vi "LEP_RV_GenerateBoardHeader.vi"(6 "Config":T1={"Enable debugging"=FALSE, "Debug Options"=0, "Use stack variables"=FALSE, "Generate serial only"=FALSE, "Generate guard code"=FALSE, "Generate Integer Only"=FALSE, "Generate C Function Calls"=TRUE, "ExpressionFolding"=TRUE, "Constant Allocation"=0, "Constant Deallocation"=0, "Build Specification ID"="", "Preprocessor symbols (define)"="", "Compiler Flags"="", "Linker Flags"="", "Mode"=1, "Optimization"=1, "Optimize for time"=FALSE, "Enable cross-module optimization"=FALSE, "Include paths"=[], "Optimize heap size"=TRUE, "Use MicroLib"=FALSE, "Debug Mode"=2, "Enable profile information"=FALSE, "Host name"="board", "Use DHCP"=TRUE, "IP address"="0.0.0.0", "Subnet mask"="", "Gateway"="0.0.0.0", "Primary DNS"="0.0.0.0", "Secondary DNS"="0.0.0.0", "MAC in target memory"=TRUE, "MAC address"="", "Console output"=1, "Target serial port"=1} {"Constant Deallocation" items=["Out of Scope", "VI End", "Application End"]; "Constant Allocation" items=["First Use", "Containing Loop", "VI Initialization", "Application Initialization"]; "Target serial port" items=["0", "1", "2", "3"]; "Console output" items=["Processor status window", "Serial port"]; "Optimization" items=["Level 0 (-O0)", "Level 1 (-O1)", "Level 2 (-O2)", "Level 3 (-O3)"]; "Mode" items=["ARM-Mode", "Thumb-Mode"]; "Debug Options" items=["Use ULINK Debugger", "Use Simulator"]; "Debug Mode" items=["Instrumented (serial port)", "Instrumented (TCP/IP)", "Non-instrumented (JTAG/USB)"]}, 8 "error in (no error)":errorcluster, 9 "Build Path":path=path "C:/ni/RealView Hello World/RealView", 11 "Rebuild":bool) -> (0 "error out":errorcluster)   [LabVIEW 2011]
doc: "Runs the embedded application on a console located in the <B>Build Path</B> directory ."
uses:
  LEP_RV_Config.ctl
  <vilib>/Platform/EmbProject/Plugins/utilities/LEP_Utilities_GetSetProjectData_U32.vi
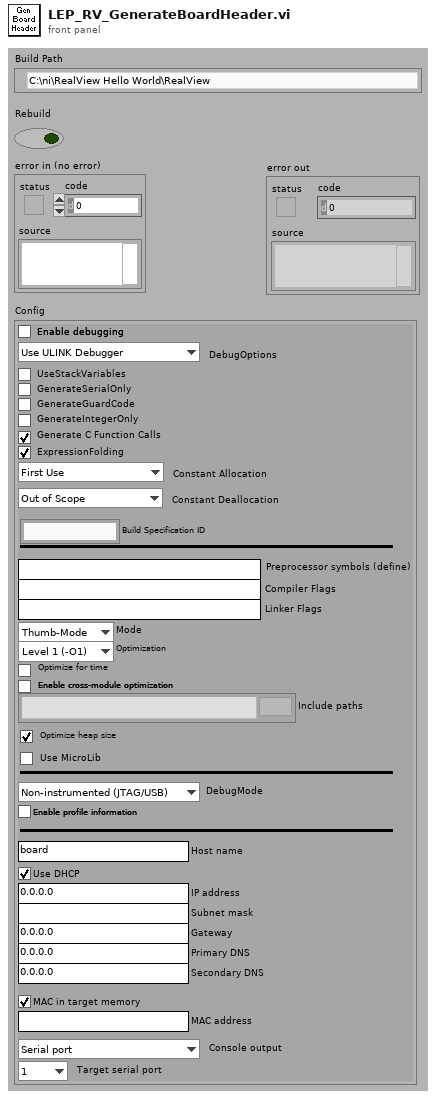
[diagram p1: front panel]
types:
  T1 = typedef "LEP_RV_Config.ctl" = cluster{"Enable debugging":bool, "Debug Options":u16, "Use stack variables":bool, "Generate serial only":bool, "Generate guard code":bool, "Generate Integer Only":bool, "Generate C Function Calls":bool, "ExpressionFolding":bool, "Constant Allocation":u16, "Constant Deallocation":u16, "Build Specification ID":string, "Preprocessor symbols (define)":string, "Compiler Flags":string, "Linker Flags":string, "Mode":u16, "Optimization":u16, "Optimize for time":bool, "Enable cross-module optimization":bool, "Include paths":path[], "Optimize heap size":bool, "Use MicroLib":bool, "Debug Mode":u16, "Enable profile information":bool, "Host name":string, "Use DHCP":bool, "IP address":string, "Subnet mask":string, "Gateway":string, "Primary DNS":string, "Secondary DNS":string, "MAC in target memory":bool, "MAC address":string, "Console output":u16, "Target serial port":u16}
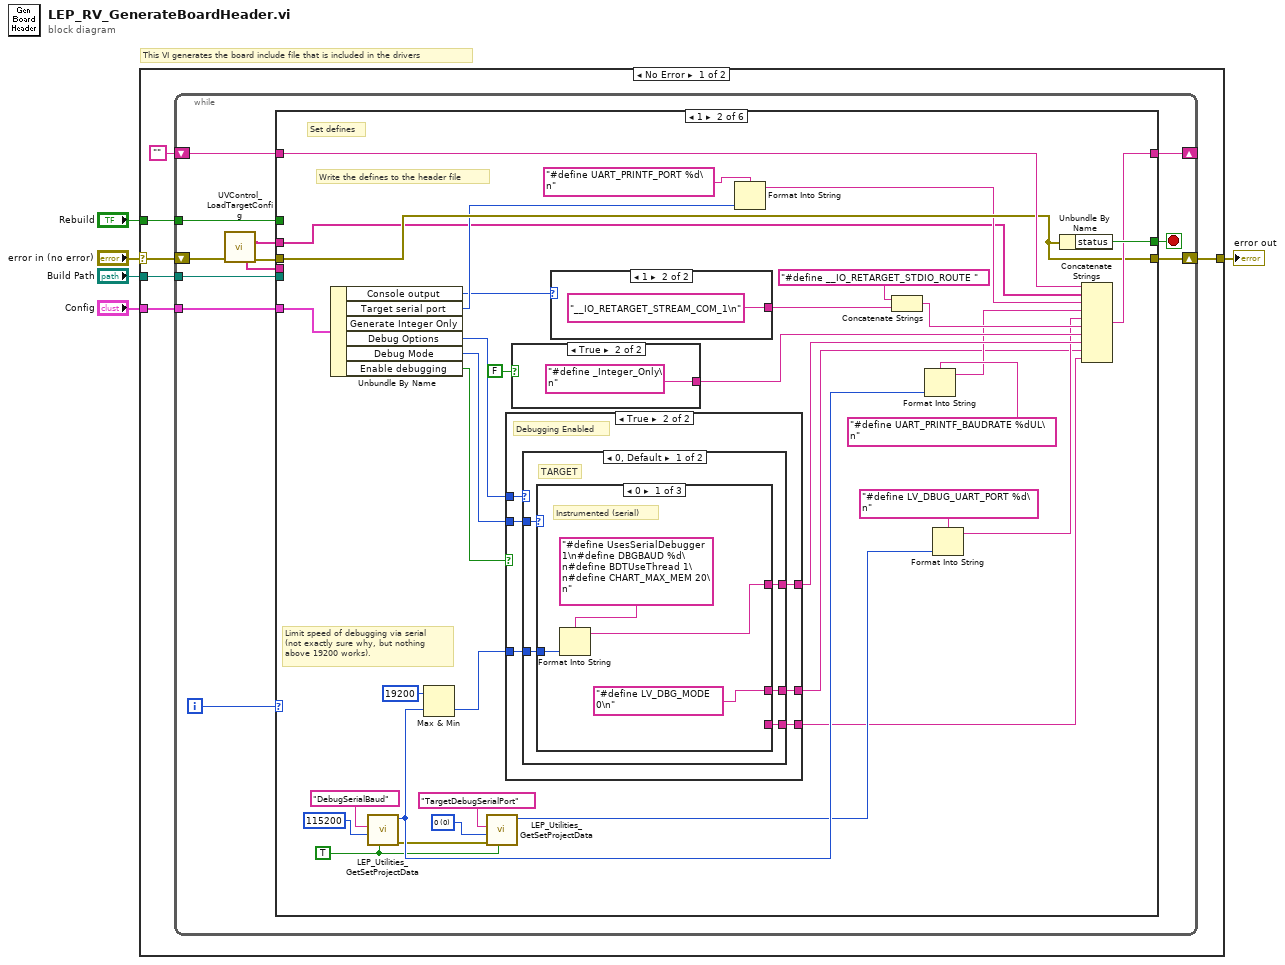
[diagram p0: block diagram]
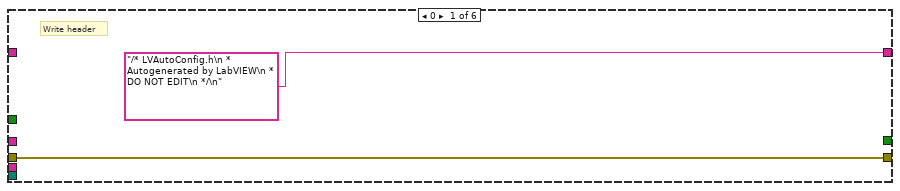
[diagram p2: hidden frame]
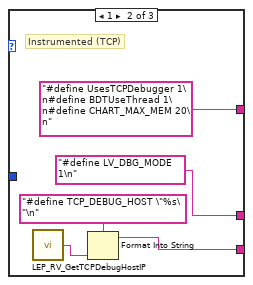
[diagram p4: hidden frame]
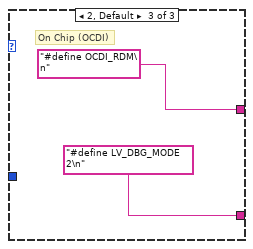
[diagram p5: hidden frame]
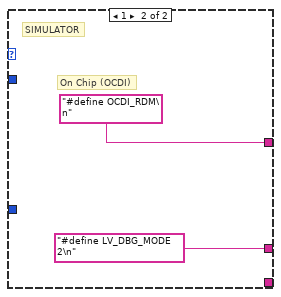
[diagram p6: hidden frame]
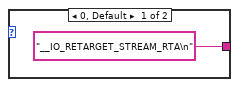
[diagram p7: hidden frame]
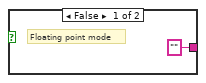
[diagram p8: hidden frame]
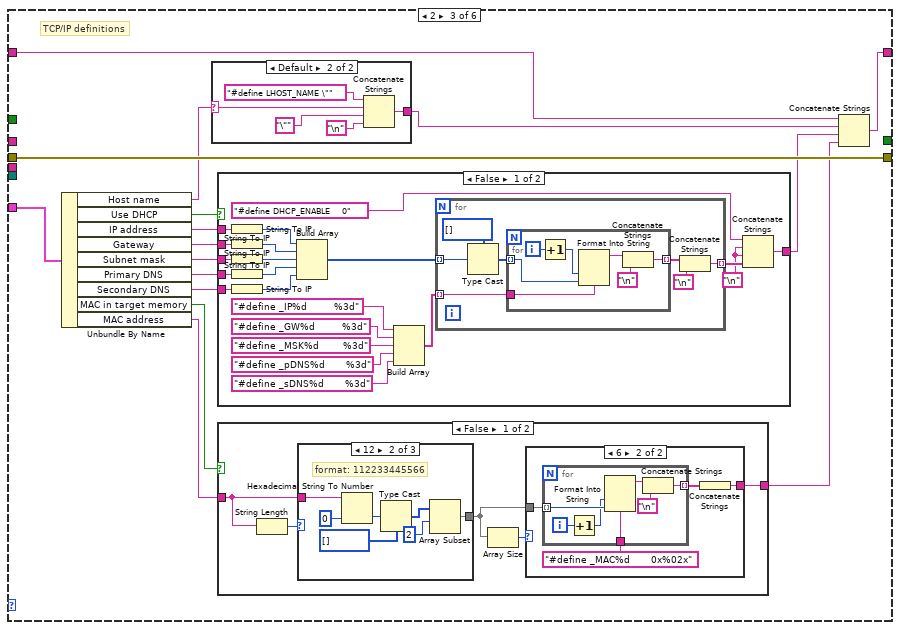
[diagram p9: hidden frame]
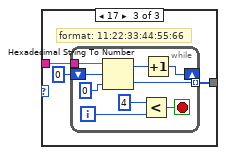
[diagram p11: hidden frame]
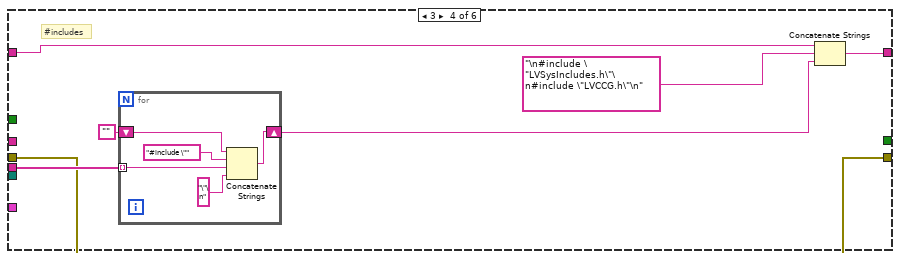
[diagram p16: hidden frame]
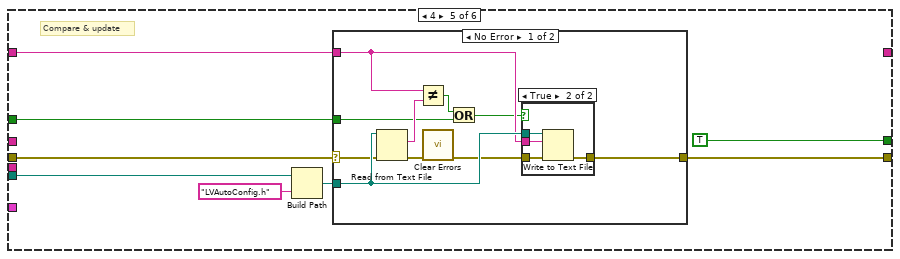
[diagram p17: hidden frame]
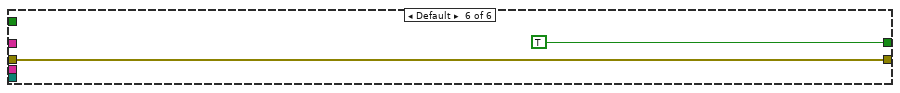
[diagram p20: hidden frame]
diagram:
  # "This VI generates the board include file that is included in the drivers"
  n1 = case shown="No Error" "error in (no error)" {
    selector: "error in (no error)" -> [w6 w218]
    tunnel: "Build Path" -> [w9 _]
    tunnel: [w11 w218] -> w3
    tunnel: "Config" -> [w10 _]
    tunnel: "Rebuild" -> [w8 _]
    frame No Error {
      n2 = while {
        tunnel: w9 -> [w23]
        shift-right: [w21] -> w11
        shift-left: w6 -> [w15]
        tunnel: w10 -> [w20]
        tunnel: w8 -> [w19]
        shift-right: [w16] -> _
        shift-left: "" -> [w17]
        i -> [w18]
        stop <- w22 stop-if-true
        n3 = call "UVControl_LoadTargetConfig.vi"("error in (no error)"=w15) -> ("Defines"=w13:string[], "Driver H Files"=w12:string[], "error out"=w14:errorcluster)  [unwired: 9 in, 3 out]
        n4 = case shown="1" w18 {
          tunnel: w23 -> [_ _ _ _ w193 _]
          tunnel: [w25 w51 w104 w184 w199 w216] -> w21
          tunnel: [_ w60 _ _ TRUE ("status") TRUE ("status")] -> w22
          tunnel: w14 -> [w25 w51 w104 w184 w195 w216]
          tunnel: w20 -> [_ w59 w103 _ _ _]
          tunnel: w19 -> [_ _ _ _ w197 _]
          tunnel: w17 -> [_ w52 w93 w182 w196 _]
          tunnel: ["/* LVAutoConfig.h\n * Autogenerated by LabVIEW\n * DO NOT EDIT\n */\n" w53 w92 w183 _ _] -> w16
          tunnel: w13 -> [_ w27 _ _ _ _]
          tunnel: w12 -> [_ _ _ w185 _ _]
          frame 0 {
            # "Write header"
          }
          frame 1 {
            w33 = u16 0 items=["0", "1", "2", "3"] ("Target serial port")
            w34 = TRUE
            # "Limit speed of debugging via serial\n(not exactly sure why, but nothing\nabove 19200 works)."
            # "Set defines"
            # "Write the defines to the header file"
            n5 = Unbundle By Name(w59) -> ("Console output"=w26:u16, "Target serial port"=w43:u16, "Debug Options"=w30:u16, "Debug Mode"=w56:u16, "Enable debugging"=w45:bool)  [unwired: 1 out]
            n6 = call-poly <vilib>:"LEP_Utilities_GetSetProjectData.vi"("access target data (F)"=w34, "data in"=u32 115200, "ItemName"="DebugSerialBaud") -> ("error out"=w37:errorcluster, "data out"=w40:u32)  [unwired: 6 in, 1 out]
            n7 = Max & Min(x=u32 19200, y=w40) -> (min(x,y)=w47:u32)  [unwired: 1 out]
            n8 = call-poly <vilib>:"LEP_Utilities_GetSetProjectData.vi"("access target data (F)"=w34, "error in"=w37, "data in"=w33, "ItemName"="TargetDebugSerialPort" ("Name")) -> ("data out"=w32:u32)  [unwired: 5 in, 2 out]
            n9 = case shown="True" w45 {
              tunnel: w56 -> [_ w63]
              tunnel: [_ w65] -> w54
              tunnel: w47 -> [_ w62]
              tunnel: [_ w64] -> w31
              tunnel: w30 -> [_ w66]
              tunnel: [_ w61] -> w29
              frame False {
                # "No Debugging"
              }
              frame True {
                # "Debugging Enabled"
                n10 = case shown="0, Default" w66 {
                  tunnel: [w69 "#define OCDI_RDM\n" ("string")] -> w65
                  tunnel: [w68 "#define LV_DBG_MODE 2\n"] -> w64
                  tunnel: w63 -> [w71 _]
                  tunnel: w62 -> [w70 _]
                  tunnel: [w67 _] -> w61
                  frame 0, Default {
                    # "TARGET"
                    n11 = case shown="0" w71 {
                      tunnel: w70 -> [w75 _ _]
                      tunnel: [w73 "#define UsesTCPDebugger 1\n#define BDTUseThread 1\n#define CHART_MAX_MEM 20\n" ("string") "#define OCDI_RDM\n" ("string")] -> w69
                      tunnel: ["#define LV_DBG_MODE 0\n" "#define LV_DBG_MODE 1\n" "#define LV_DBG_MODE 2\n"] -> w68
                      tunnel: [_ w77 _] -> w67
                      frame 0 {
                        # "Instrumented (serial)"
                        n12 = Format Into String(format string="#define UsesSerialDebugger 1\n#define DBGBAUD %d\n#define BDTUseThread 1\n#define CHART_MAX_MEM 20\n" ("string"), w75) -> (resulting string=w73:string)  [unwired: 2 in, 1 out]
                      }
                      frame 1 {
                        # "Instrumented (TCP)"
                        n13 = call "LEP_RV_GetTCPDebugHostIP.vi"() -> ("IP Address"=w76:string)  [unwired: 1 in]
                        n14 = Format Into String(format string="#define TCP_DEBUG_HOST \"%s\"\n", w76) -> (resulting string=w77:string)  [unwired: 2 in, 1 out]
                      }
                      frame 2, Default {
                        # "On Chip (OCDI)"
                      }
                    }
                  }
                  frame 1 {
                    # "On Chip (OCDI)"
                    # "SIMULATOR"
                  }
                }
              }
            }
            n15 = case shown="True" FALSE {
              tunnel: ["" ("string") "#define _Integer_Only\n" ("string")] -> w55
              frame False {
                # "Floating point mode"
              }
              frame True {
              }
            }
            n16 = case shown="1" w26 {
              tunnel: ["__IO_RETARGET_STREAM_RTA\n" "__IO_RETARGET_STREAM_COM_1\n"] -> w46
              frame 0, Default {
              }
              frame 1 {
              }
            }
            n17 = Format Into String(format string="#define UART_PRINTF_PORT %d\n", w43) -> (resulting string=w42:string)  [unwired: 2 in, 1 out]
            n18 = Concatenate Strings("#define __IO_RETARGET_STDIO_ROUTE " ("string"), w46) -> (w57:string)
            n19 = Format Into String(format string="#define UART_PRINTF_BAUDRATE %dUL\n", w40) -> (resulting string=w39:string)  [unwired: 2 in, 1 out]
            n20 = Format Into String(format string="#define LV_DBUG_UART_PORT %d\n", w32) -> (resulting string=w35:string)  [unwired: 2 in, 1 out]
            n21 = Unbundle By Name(w51) -> ("status"=w60:bool)
            n22 = Concatenate Strings(w52, w27, w42, w39, w35, w57, w55, w54, w31, w29) -> (w53:string)
          }
          frame 2 {
            # "TCP/IP definitions"
            n23 = Unbundle By Name(w103) -> ("Host name"=w102:string, "Use DHCP"=w100:bool, "IP address"=w99:string, "Gateway"=w98:string, "Subnet mask"=w97:string, "Primary DNS"=w96:string, "Secondary DNS"=w95:string, "MAC in target memory"=w91:bool, "MAC address"=w90:string)
            n24 = case shown="Default" w102 {
              selector: w102 -> [_ w178]
              tunnel: [_ w176] -> w101
              frame "" {
              }
              frame Default {
                n25 = Concatenate Strings("#define LHOST_NAME \"" ("string"), w178, "\"", "\n") -> (w176:string)
              }
            }
            n26 = case shown="False" w100 {
              tunnel: [w141 _] -> w94
              tunnel: w99 -> [w160 _]
              tunnel: w98 -> [w156 _]
              tunnel: w97 -> [w159 _]
              tunnel: w96 -> [w158 _]
              tunnel: w95 -> [w157 _]
              frame False {
                w140 = "\n"
                n27 = String To IP(1:w160) -> (0:w155:u32)
                n28 = String To IP(1:w156) -> (0:w154:u32)
                n29 = String To IP(1:w159) -> (0:w153:u32)
                n30 = String To IP(1:w158) -> (0:w151:u32)
                n31 = String To IP(1:w157) -> (0:w152:u32)
                n32 = Build Array(w155, w154, w153, w151, w152) -> (w145:u32[])
                n33 = Build Array("#define _IP%d         %3d", "#define _GW%d         %3d", "#define _MSK%d        %3d", "#define _pDNS%d       %3d", "#define _sDNS%d       %3d") -> (w144:string[])
                n34 = for {
                  tunnel: w145 -> [w167] mode=indexing
                  tunnel: w144 -> [w165] mode=indexing
                  tunnel: [w162] -> w143 mode=indexing
                  n35 = Type Cast(type=u8[] [], x=w167) -> (*(type *) &x=w164:u8[])
                  n36 = for {
                    tunnel: w165 -> [w174]
                    tunnel: w164 -> [w172] mode=indexing
                    tunnel: [w170] -> w163 mode=indexing
                    i -> [w173]
                    n37 = Increment(x=w173) -> (x+1=w168:i32)
                    n38 = Format Into String(format string=w174, w168, w172) -> (resulting string=w171:string)  [unwired: 2 in, 1 out]
                    n39 = Concatenate Strings(w171, "\n") -> (w170:string)
                  }
                  n40 = Concatenate Strings(w163, "\n") -> (w162:string)
                }
                n41 = Concatenate Strings("#define DHCP_ENABLE    0", w140, w140, w143) -> (w141:string)
              }
              frame True {
              }
            }
            n42 = case shown="False" w91 {
              tunnel: w90 -> [w106 _]
              tunnel: [w105 _] -> w89
              frame False {
                n43 = String Length(string=w106) -> (length=w108:i32)
                n44 = case shown="12" w108 {
                  tunnel: [_ w111 w118] -> w109
                  tunnel: w106 -> [_ w116 w117]
                  frame Default {
                    # "Is this a MAC address ?\n\nThese formats are allowed:\nxx:xx:xx:xx:xx:xx\nxx xx xx xx xx xx\nxxxxxxxxxxxx"
                  }
                  frame 12 {
                    # "format: 112233445566"
                    n45 = Hexadecimal String To Number(string=w116, default (0uL)=u64 0 ("default (0 U32)")) -> (number=w114:u64)  [unwired: 1 in, 1 out]
                    n46 = Type Cast(type=u8[] [], x=w114) -> (*(type *) &x=w112:u8[])
                    n47 = Array Subset(array=w112, index=2) -> (w111:u8[])  [unwired: 1 in]
                  }
                  frame 17 {
                    # "format: 11:22:33:44:55:66"
                    n48 = while {
                      tunnel: w117 -> [w127]
                      shift-right: [w124] -> _
                      shift-left: 0 ("offset") -> [w128]
                      tunnel: [w126] -> w118 mode=indexing
                      i -> [w122]
                      stop <- w120 stop-if-true
                      n49 = Hexadecimal String To Number(string=w127, offset=w128, default (0uL)=u8 0) -> (offset past number=w121:i32, number=w126:u8)
                      n50 = Less?(x=4 ("y"), y=w122) -> (x < y?=w120:bool)
                      n51 = Increment(x=w121) -> (x+1=w124:i32)
                    }
                  }
                }
                n52 = Array Size(array=w109) -> (size(s)=w107:i32)
                n53 = case shown="6" w107 {
                  tunnel: w109 -> [_ w132]
                  tunnel: [_ w129] -> w105
                  frame Default {
                  }
                  frame 6 {
                    n54 = for {
                      tunnel: w132 -> [w138] mode=indexing
                      tunnel: "#define _MAC%d       0x%02x" -> [w137]
                      tunnel: [w135] -> w130 mode=indexing
                      i -> [w139]
                      n55 = Increment(x=w139) -> (x+1=w133:i32)
                      n56 = Format Into String(format string=w137, w133, w138) -> (resulting string=w136:string)  [unwired: 2 in, 1 out]
                      n57 = Concatenate Strings(w136, "\n") -> (w135:string)
                    }
                    n58 = Concatenate Strings(w130) -> (w129:string)
                  }
                }
              }
              frame True {
              }
            }
            n59 = Concatenate Strings(w93, w101, w94, w89) -> (w92:string)
          }
          frame 3 {
            # "#includes"
            n60 = for {
              tunnel: w185 -> [w190] mode=indexing
              shift-right: [w188] -> w181
              shift-left: "" -> [w187]
              n61 = Concatenate Strings(w187, "#include \"" ("string"), w190, "\"\n" ("string")) -> (w188:string)
            }
            n62 = Concatenate Strings(w182, "\n#include \"LVSysIncludes.h\"\n#include \"LVCCG.h\"\n", w181) -> (w183:string)
          }
          frame 4 {
            # "Compare & update"
            n63 = Build Path(base path=w193, name or relative path="LVAutoConfig.h") -> (appended path=w192:path)
            n64 = case shown="No Error" w195 {
              selector: w195 -> [w207 w215]
              tunnel: [w209 w215] -> w199
              tunnel: w192 -> [w208 _]
              tunnel: w197 -> [w200 _]
              tunnel: w196 -> [w203 _]
              frame No Error {
                n65 = Read from Text File(file (use dialog)=w208, error in=w207) -> (text=w206:string, error out=w205:errorcluster)  [unwired: 2 in, 2 out]
                n66 = Not Equal?(x=w203, y=w206) -> (x != y?=w201:bool)
                n67 = call <vilib>:"Clear Errors.vi"("error in (no error)"=w205) -> ("error out"=w204:errorcluster)  [unwired: 6 in]
                n68 = Or(x=w201, y=w200) -> (x .or. y?=w202:bool)
                n69 = case shown="True" w202 {
                  tunnel: w208 -> [_ w212]
                  tunnel: w204 -> [w210 w214]
                  tunnel: [w210 w213] -> w209
                  tunnel: w203 -> [_ w211]
                  frame False {
                  }
                  frame True {
                    n70 = Write to Text File(file (use dialog)=w212, text=w211, error in=w214) -> (error out=w213:errorcluster)  [unwired: 1 in, 2 out]
                  }
                }
              }
              frame Error {
              }
            }
          }
          frame Default {
          }
        }
      }
    }
    frame Error {
    }
  }
  "error out" <- w3
